vi "Check Table Existence.vi"(8 "error in (no error)":errorcluster, 10 "element":string, 11 "Refnum in":T1) -> (0 "error out":errorcluster, 3 "Table Exist?":bool)   [LabVIEW 2018]
doc: "Returns true if specified table exists"
uses:
  <vilib>/addons/database/Connection.llb/Conn ObjectReference.ctl
  <vilib>/addons/database/NI_Database_API.lvlib
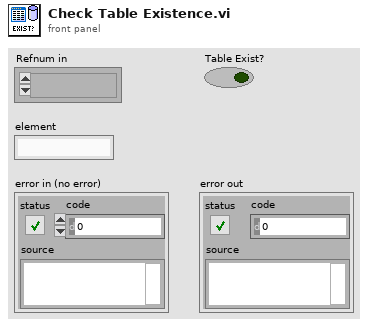
[diagram p1: front panel]
types:
  T1 = typedef "NI_Database_API.lvlib/Conn ObjectReference.ctl" = refnum<k1>
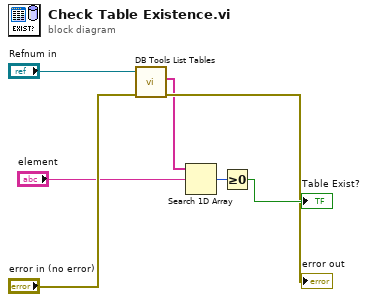
[diagram p0: block diagram]
diagram:
  n1 = call <vilib>:"DB Tools List Tables.vi"("error in (no error)"="error in (no error)", "connection reference"="Refnum in") -> ("error out"=→"error out":errorcluster, "tables"=w2:string[])  [unwired: 3 in, 1 out]
  n2 = Search 1D Array(1D array=w2, element="element") -> (index of element=w6:i32)  [unwired: 1 in]
  n3 = Greater Or Equal To 0?(x=w6) -> (x >= 0?=→"Table Exist?":bool)
